vi "RT_Main.vi"(8 "ErrorIn":errorcluster, 11 "ClusterIn":T1={"MainQ"=refnum, "User"={"Lvl"=enum."Admin", "Pwd"=""}, "Stat"={"SysState"=enum."Init"}, "Paths"={"CfgFile"=path "", "LogFolder"=path "", "LogFile"=path ""}, "HW"={"HW?"=FALSE, "HWMode"=enum."HW_Init", "Refs"={"Visa"="GPIB0::2::INSTR"}}, "RTConfig"={"Arm"=FALSE, "Number"=0.0, "String"=""}}) -> (0 "ErrorOut":errorcluster, 3 "ClusterOut":T1={"MainQ"=refnum, "User"={"Lvl"=enum."Admin", "Pwd"=""}, "Stat"={"SysState"=enum."Init"}, "Paths"={"CfgFile"=path "", "LogFolder"=path "", "LogFile"=path ""}, "HW"={"HW?"=FALSE, "HWMode"=enum."HW_Init", "Refs"={"Visa"="GPIB0::2::INSTR"}}, "RTConfig"={"Arm"=FALSE, "Number"=0.0, "String"=""}})   [LabVIEW 2018]
doc: "This is the main application VI and is a good framework to begin all applications with. See block diagram for detailed documentation.\n\n\nCopyright © 2011 Epimedia, Inc. All Rights Reserved.\n\nThe Epimedia Application Library is Copyright © 2009-2011 Epimedia, Inc. \nAll Rights Reserved. Used under license."
uses:
  Controls/UserLevelEnum_RT.ctl
  Queue/RTMainQueueElements.ctl
  Queue/HWQueueElements.ctl
  Queue/HyperVisor.ctl
  Controls/SystemStateEnum_RT.ctl
  Controls/Enums/RT_WinRead_Enum_RT.ctl
  Controls/Clusts/StreamClust.ctl
  <resource>/objmgr/ni.dex.rc
  Controls/Enums/WriteStream_RT.ctl
  Queue/MainQueueElements.ctl
  Controls/RT_Config.ctl
  Controls/HWCluster_RT.ctl
  Controls/HWRefsCluster_RT.ctl
  Controls/MasterCluster_RT.ctl
  Controls/PathsCluster_RT.ctl
  Controls/UserCluster_RT.ctl
  Controls/SystemStatusCluster_RT.ctl
panel:
  out "30 Second Time":string
  out "CPU":dbl
  in  "ReInitHW":bool
  in  "ErrorIn":errorcluster
  out "Time":timestamp caption="Current Date/Time" format="%<%H:%M:%S%1u\n%m/%d/%Y>T"
  in  "Start":bool
  in  "Exit":bool
  in  "Stop":bool
  # "Copyright © 2011 Epimedia, Inc. All Rights Reserved.\n\nThe Epimedia Application Library is Copyright © 2009-2011 Epimedia, Inc. \nAll Rights Reserved. Used under license."
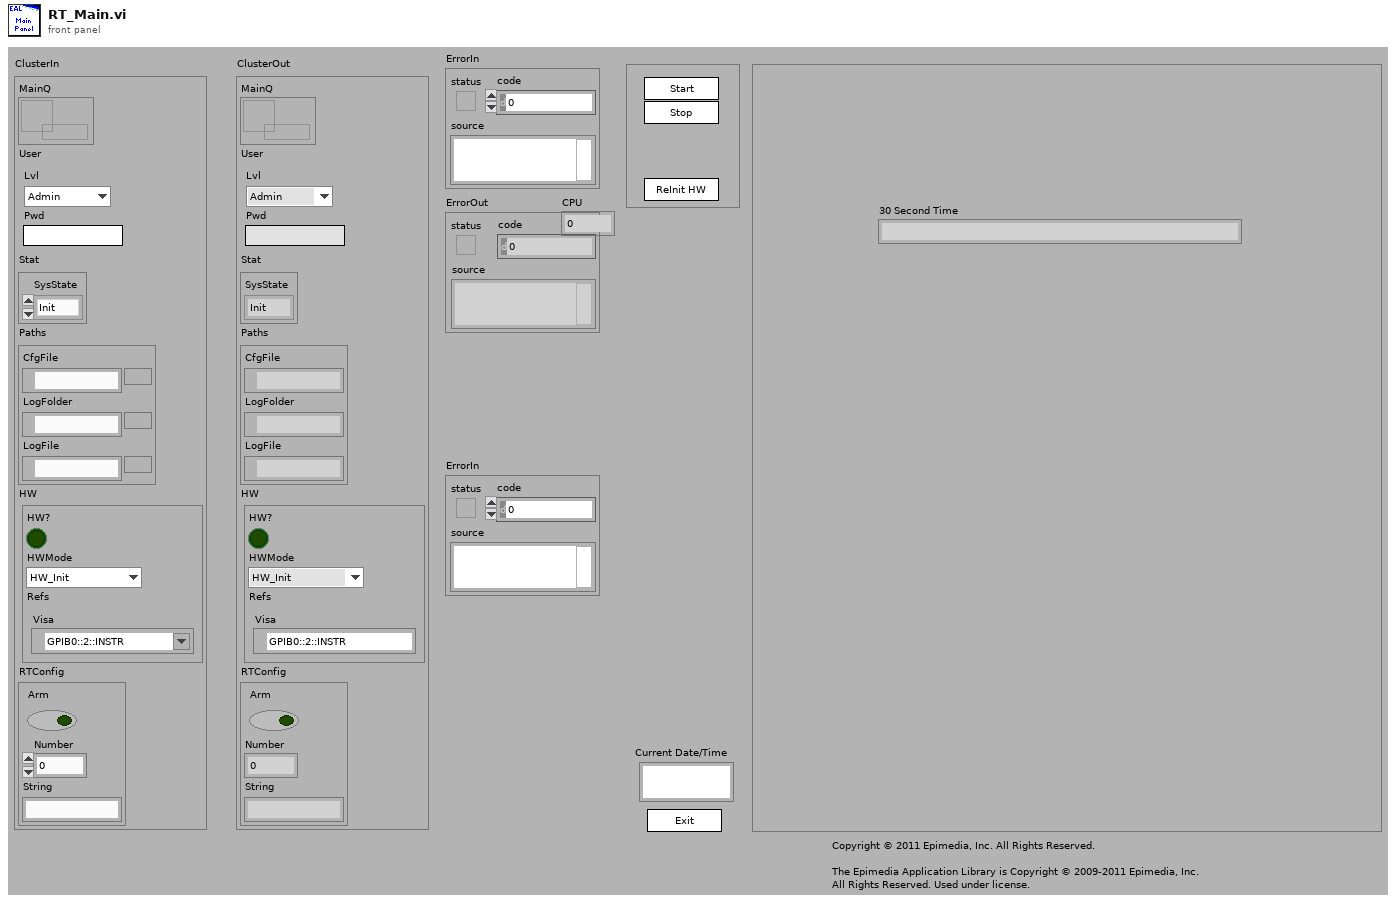
[diagram p1: front panel]
types:
  T1 = typedef "MasterCluster_RT.ctl" = cluster{"MainQ":refnum<queue>, "User":T2, "Stat":T4, "Paths":T6, "HW":T7, "RTConfig":T10}
  T2 = typedef "UserCluster_RT.ctl" = cluster{"Lvl":T3, "Pwd":string}
  T3 = typedef "UserLevelEnum_RT.ctl" = enum16{"Admin", "Operator"}
  T4 = typedef "SystemStatusCluster_RT.ctl" = cluster{"SysState":T5}
  T5 = typedef "SystemStateEnum_RT.ctl" = enum16{"Init", "Idle", "Running", "Error", "Exit"}
  T6 = typedef "PathsCluster_RT.ctl" = cluster{"CfgFile":path, "LogFolder":path, "LogFile":path}
  T7 = typedef "HWCluster_RT.ctl" = cluster{"HW?":bool, "HWMode":T8, "Refs":T9}
  T8 = typedef "HWQueueElements.ctl" = enum16{"HW_Init", "HW_UpdtCfg", "HW_Start", "HW_Pause", "HW_Run", "HW_Cls", "HW_Exit"}
  T9 = typedef "HWRefsCluster_RT.ctl" = cluster{"Visa":refnum<visa-resource-name>}
  T10 = typedef "RT_Config.ctl" = cluster{"Arm":bool, "Number":dbl, "String":string}
  T11 = typedef "WriteStream_RT.ctl" = enum16{"CreateWrtr", "SendStrm"}
  T12 = enum16{"open", "replace", "create", "open or create", "replace or create", "replace or create with confirmation"}
  T13 = typedef "RT_WinRead_Enum_RT.ctl" = enum16{"Init", "Read", "AUTO_Poll"}
  T14 = typedef "HyperVisor.ctl" = cluster{"TimeOut":dbl, string, "Data":variant, "StopHpvsr":bool}
  T15 = typedef "RTMainQueueElements.ctl" = enum16{"RTMain_InitQ", "RTMain_InitSW", "RTMain_InitCtrls", "RTMain_ReInitHW", "RTMain_FromStream", "RTMain_StrtHWLp", "RTMain_UpdtHWClstr", "RTMain_Start", "RTMain_Stop", "RTMain_Error", "RTMain_Config", "RTMain_Exit"}
  T16 = typedef "HWQueueElements.ctl" = enum16{"RTHW_Init", "RTHW_UpdtCfg", "RTHW_Start", "RTHW_Pause", "RTHW_Run", "RTHW_Cls", "RTHW_Exit"}
  T17 = typedef "MasterCluster.ctl" = cluster{"Admin":T18, "RTConfig":T10, "SMS":T20, "FPGA":T21, "Config":T23, "Stat":T33, "Alarm":T35}
  T18 = typedef "AdminCluster.ctl" = cluster{"Lvl":T19, "Pwd":string}
  T19 = typedef "UserLevelEnum.ctl" = enum16{"Admin", "Operator"}
  T20 = typedef "SMSDataCluster.ctl" = cluster{"Enbl?":bool, "Addr":string[]}
  T21 = typedef "FPGA_Config_Clust.ctl" = cluster{"Target":T22, "Channel":T22, "Ref1":refnum<k20>, "Ref2":refnum<k20>}
  T22 = typedef "TargetNumber.ctl" = enum16{"1", "2", "3", "4"}
  T23 = typedef "Config_Clust.ctl" = cluster{"UsrCfg":T24, "FP_User":T26}
  T24 = typedef "UserConfig.ctl" = cluster{"Paths":T25, "SampleRate":dbl}
  T25 = typedef "PathsCluster.ctl" = cluster{"CfgFile":path, "LogFolder":path, "LogFile":path, "NAS path":path, "ThreshFile":path, "RedunFolder":path}
  T26 = typedef "FrontPanel_UserConfig.ctl" = cluster{"#NoiseSums":u32, "Max_df":u32, "AvgAvg":bool, "#Avg":u16, "AutoCenter":bool, "Inclin":T27, "1":T28, "2":T28, "3":T28, "4":T28, "Target to Probe":T22, "SNR_Thresh":dbl, "Paths":T25, "Connex_Location":string, "SimulateFPGA":bool}
  T27 = typedef "Inclinometer_User_Cfg.ctl" = cluster{"Vmin":dbl, "Vmax":dbl, "Angle_min":dbl, "Angle_max":dbl, "Offset":dbl, "Pos_Neg":bool}
  T28 = typedef "FP_UserTargetConfig.ctl" = cluster{"Cal_":T29, "Beac":T29, "Scale":T30, "Offset":fxp<+/-,16,16>, "Scale_Noise":fxp<+/-,30,30>, "Scale_Step1":fxp<+/-,17,17>, "Scale_In_RT":ext, "ScaleMeas":fxp<+/-,16,1>, "FreqsToRemove":i32[], "Width":i32[], "ScaleMeasEnum":T31, "FilterEnab":T32}
  T29 = typedef "FreqShift.ctl" = cluster{"Fine":dbl, "Coarse_":dbl}
  T30 = typedef "FPGA_Scale.ctl" = cluster{"Step4":fxp<+/-,23,23>, "Step5":fxp<+/-,23,23>, "Step6":fxp<+/-,23,23>, "Step7":fxp<+/-,23,23>}
  T31 = typedef "ScaleMeasure.ctl" = enum16{"1", "10", "50", "42"}
  T32 = typedef "FilterEnableRadio.ctl" = enum32{"None", "Step 1", "Frequency Shift", "Step 4", "Step 5", "Step 6", "Step 7"}
  T33 = typedef "SystemStatusCluster.ctl" = cluster{"SysState":T34, "TrackRate":bool, "AutoCentr":bool}
  T34 = typedef "SystemStateEnum.ctl" = enum16{"Init", "Idle", "Running", "System Fault", "System Error", "Exit"}
  T35 = typedef "AlarmSettingsClust.ctl" = cluster{"TC13":T36, "AI1":T36, "AI2":T36, "AI3":T36, "AI4":T36, "AI5":T36, "AI6":T36, "AI18":T36, "AI19":T36, "TE1":T36, "TE2":T36, "TE3":T36, "ADAM1":T36, "ADAM2":T36, "ADAM3":T36, "ADAM4":T36, "72CoBeacFreq":T36, "72CoCalFreq":T36, "84CoBeacFreq":T36, "84CoCalFreq":T36, "72Co_CalTonePwr":T36, "72X_CalTonePwr":T36, "84Co_CalTonePwr":T36, "84X_CalTonePwr":T36}
  T36 = typedef "AlarmThresh_OneChan.ctl" = cluster{"Enbl":bool, "ErrsAndWarns":cluster{dbl, dbl, dbl, dbl}}
  T37 = typedef "MainQueueElements.ctl" = enum16{"Spvsr_InitQ", "Spvsr_RfrshPnl", "Spvsr_InitSW", "Spvsr_InitCtrls", "Spvsr_Cursors", "Spvsr_StrtHWLp", "Spvsr_Stop", "Spvsr_NewData", "Spvsr_ScaleGraphs", "Spvsr_Error", "Spvsr_About", "Spvsr_Config", "Spvsr_FPConfig", "Spvsr_AlarmCfg", "Spvsr_DigitzOffs", "FP_AO_ctrl", "Spvsr_RestartWarn", "Spvsr_AutoCenter", "Spvsr_TrackRate", "Spvsr_ChkTime", "Spvsr_Admin", "Spvsr_Exit"}
  T38 = typedef "NI_Real-Time Target Support.lvlib/RT CPU Load.ctl" = cluster{"Total (%)":dbl, "Time Critical (%)":dbl, "Timed Structures (%)":dbl, "High (%)":dbl, "Above Normal (%)":dbl, "Normal (%)":dbl, "Background (%)":dbl, "Idle (%)":dbl, "ISR (%)":dbl}
  T39 = typedef "StreamClust.ctl" = cluster{u16, variant}
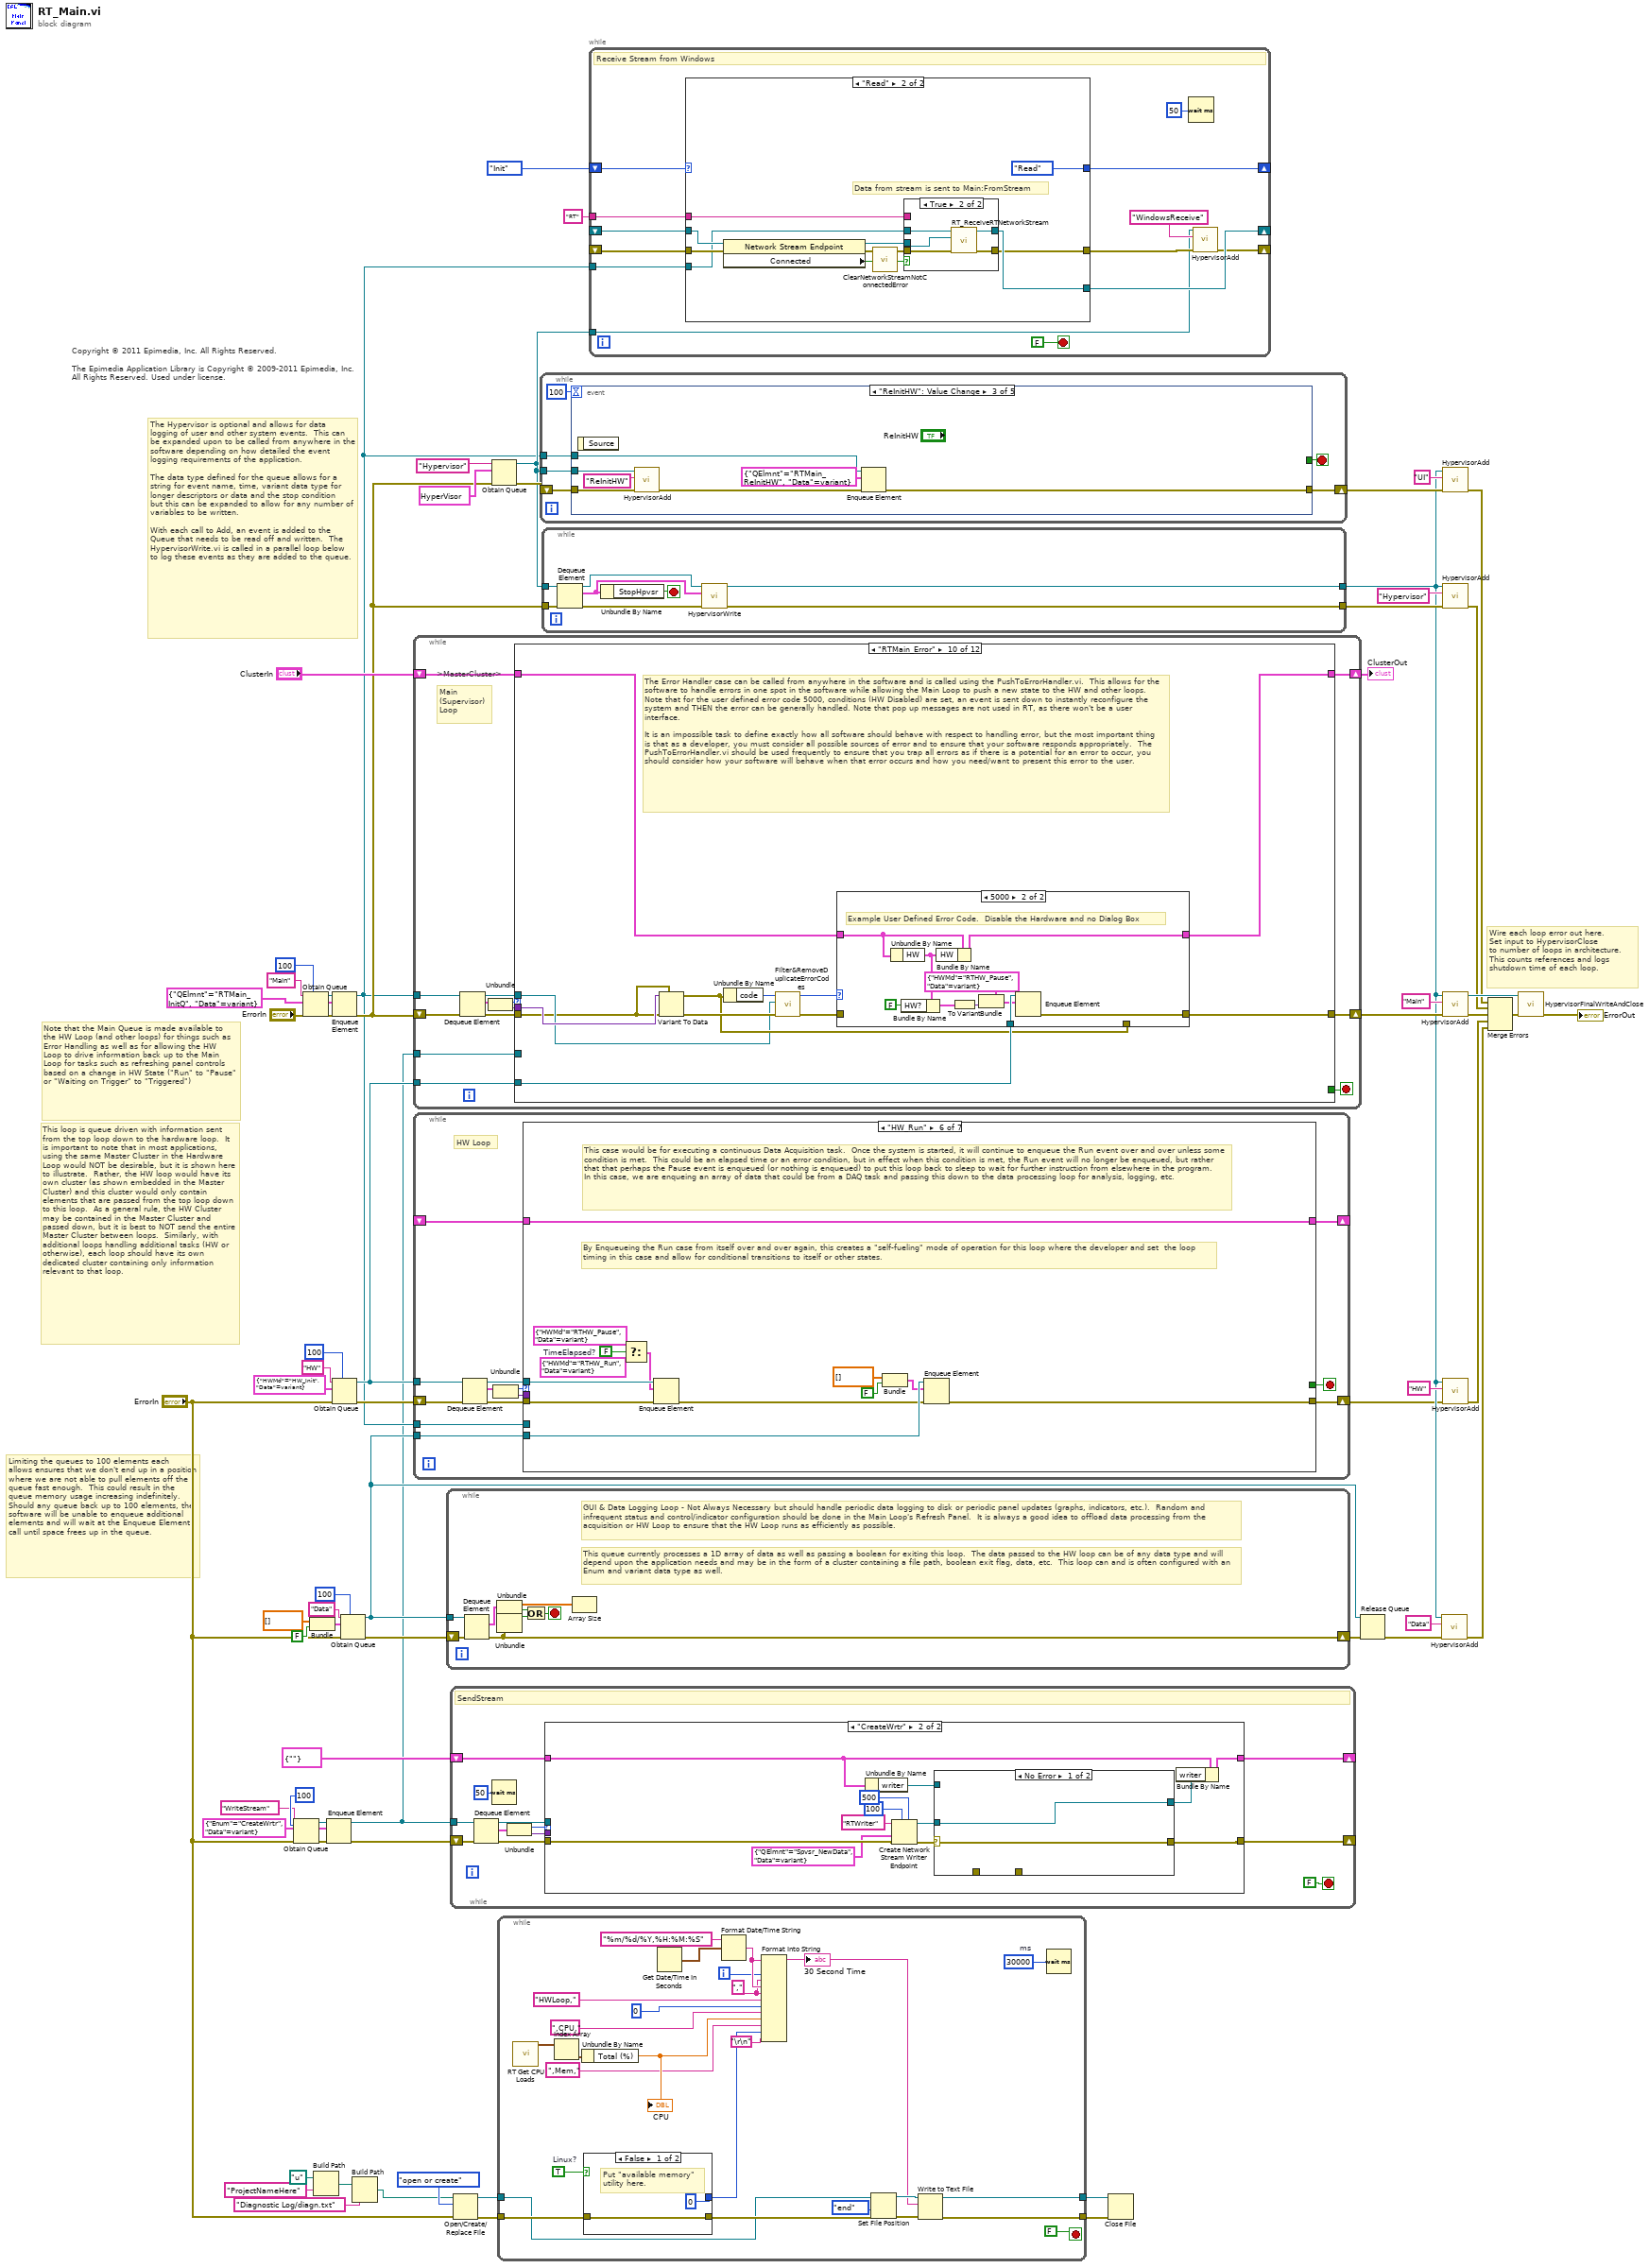
[diagram p0: block diagram]
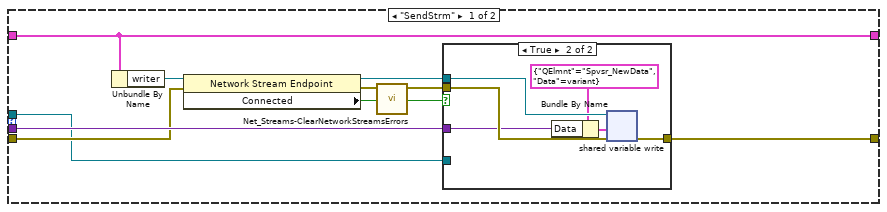
[diagram p2: hidden frame]
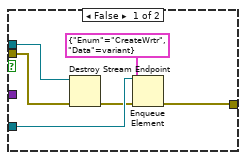
[diagram p3: hidden frame]
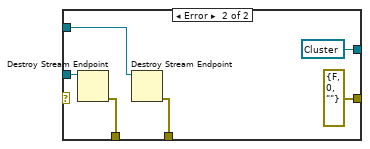
[diagram p4: hidden frame]
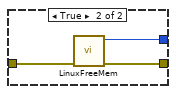
[diagram p5: hidden frame]
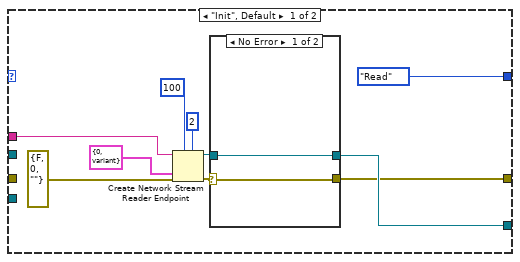
[diagram p6: hidden frame]
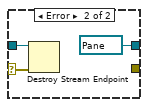
[diagram p7: hidden frame]
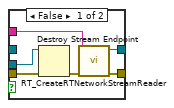
[diagram p8: hidden frame]
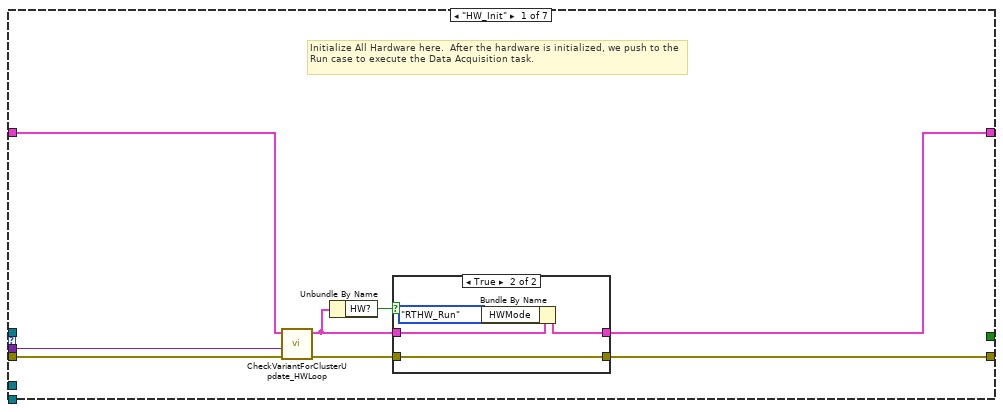
[diagram p9: hidden frame]
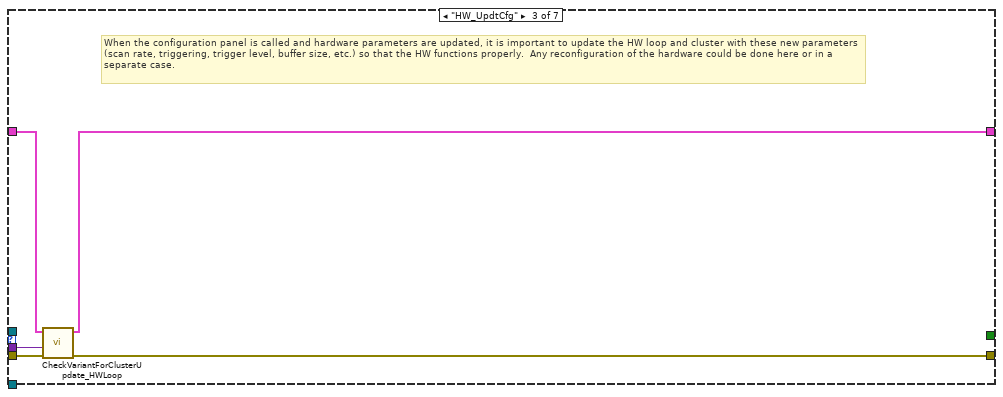
[diagram p12: hidden frame]
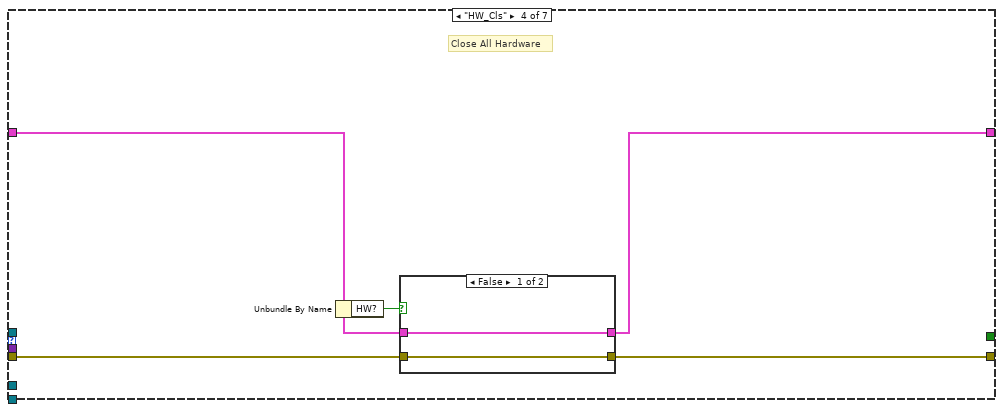
[diagram p13: hidden frame]
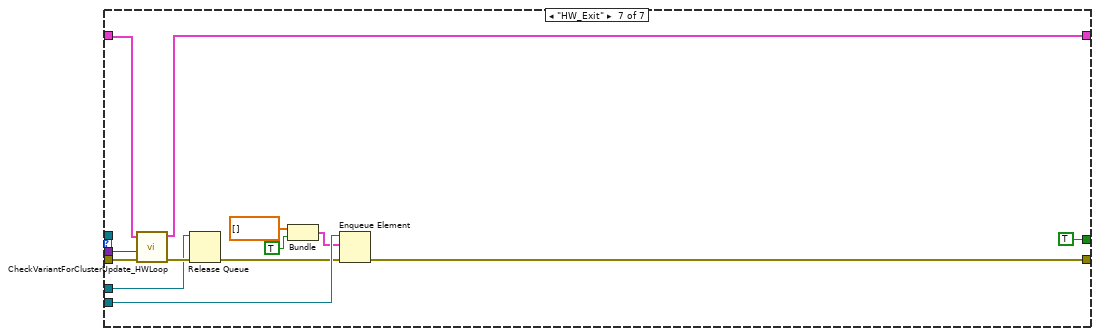
[diagram p16: hidden frame]
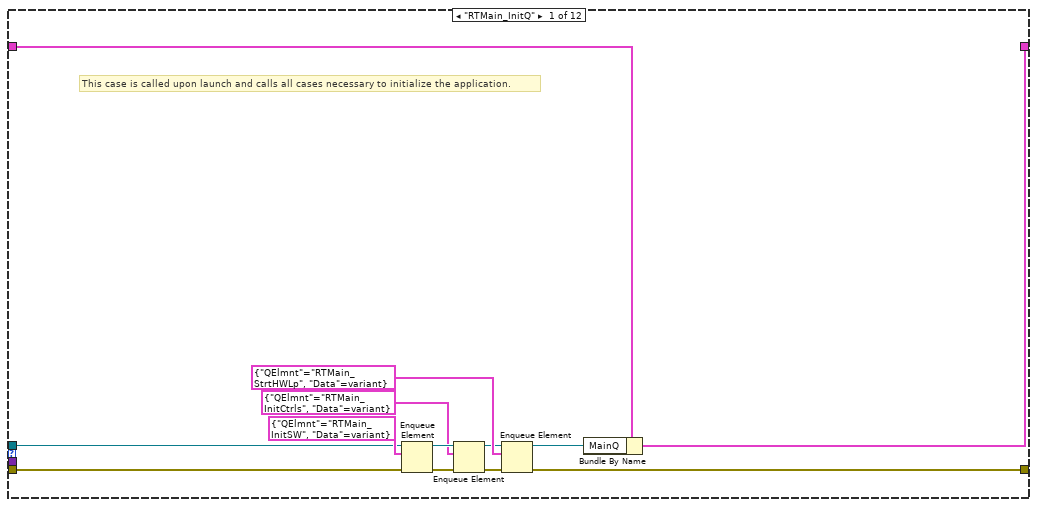
[diagram p17: hidden frame]
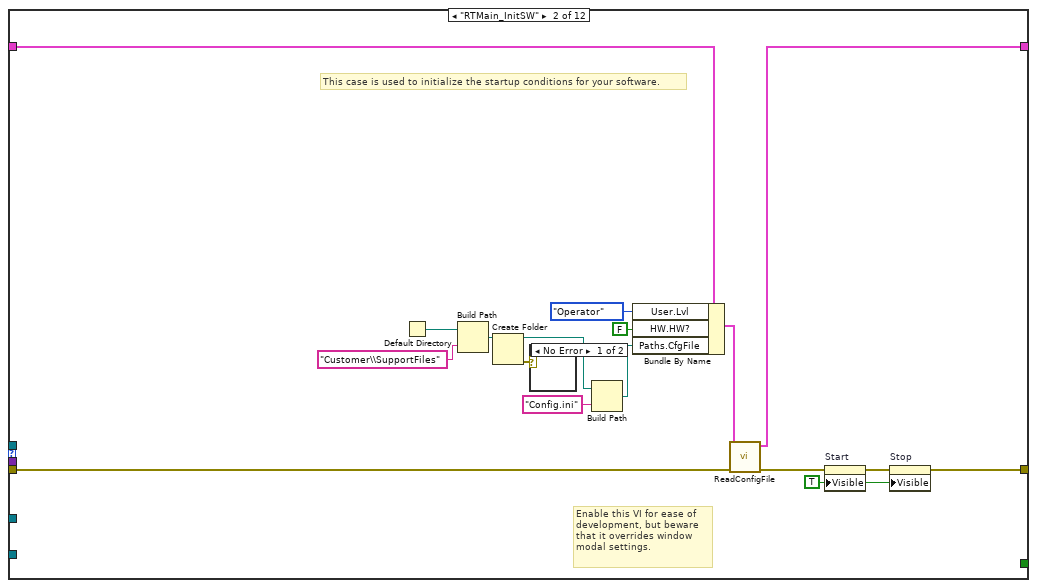
[diagram p18: hidden frame]
diagram:
  w12 = cluster{"Enum":T11, "Data":variant} {"Enum"=enum."CreateWrtr", "Data"=variant} ("output cluster")
  w62 = cluster{"QElmnt":T15, "Data":variant} {"QElmnt"=enum."RTMain_InitQ", "Data"=variant} ("Cluster")
  # "Note that the Main Queue is made available to the HW Loop (and other loops) for things such as Error Handling as well as for allowing the HW Loop to drive information back up to the Main Loop for tasks such as refreshing panel controls  based on a change in HW State (\"Run\" to \"Pause\" or \"Waiting on Trigger\" to \"Triggered\")"
  # "Limiting the queues to 100 elements each allows ensures that we don't end up in a position where we are not able to pull elements off the queue fast enough.  This could result in the queue memory usage increasing indefinitely.  Should any queue back up to 100 elements, the software will be unable to enqueue additional elements and will wait at the Enqueue Element call until space frees up in the queue."
  # "Wire each loop error out here.\nSet input to HypervisorClose\nto number of loops in architecture.\nThis counts references and logs\nshutdown time of each loop."
  # "The Hypervisor is optional and allows for data logging of user and other system events.  This can be expanded upon to be called from anywhere in the software depending on how detailed the event logging requirements of the application.\n\nThe data type defined for the queue allows for a string for event name, time, variant data type for longer descriptors or data and the stop condition but this can be expanded to allow for any number of variables to be written.\n\nWith each call to Add, an event is added to the Queue that needs to be read off and written.  The HypervisorWrite.vi is called in a parallel loop below to log these events as they are added to the queue."
  # "This loop is queue driven with information sent from the top loop down to the hardware loop.  It is important to note that in most applications, using the same Master Cluster in the Hardware Loop would NOT be desirable, but it is shown here to illustrate.  Rather, the HW loop would have its own cluster (as shown embedded in the Master Cluster) and this cluster would only contain elements that are passed from the top loop down to this loop.  As a general rule, the HW Cluster may be contained in the Master Cluster and passed down, but it is best to NOT send the entire Master Cluster between loops.  Similarly, with additional loops handling additional tasks (HW or otherwise), each loop should have its own dedicated cluster containing only information relevant to that loop."
  # "Copyright © 2011 Epimedia, Inc. All Rights Reserved.\n\nThe Epimedia Application Library is Copyright © 2009-2011 Epimedia, Inc. \nAll Rights Reserved. Used under license."
  n1 = Obtain Queue(max queue size (-1, unlimited)=100, name (unnamed)="WriteStream", element data type=w12, error in (no error)="ErrorIn") -> (queue out=w15:refnum<queue>, error out=w11:errorcluster)  [unwired: 1 in, 1 out]
  n2 = Obtain Queue(max queue size (-1, unlimited)=100, name (unnamed)="Main", element data type=w62, error in (no error)="ErrorIn") -> (queue out=w65:refnum<queue>, error out=w66:errorcluster)  [unwired: 1 in, 1 out]
  n3 = Bundle(dbl[] [], FALSE) -> (w27:cluster{dbl[], bool})  [unwired: 1 in]
  n4 = Build Path(base path=path "u", name or relative path="ProjectNameHere") -> (appended path=w3:path)
  n5 = Enqueue Element(queue=w15, element=w12, error in (no error)=w11) -> (queue out=w7:refnum<queue>, error out=w10:errorcluster)  [unwired: 1 in, 1 out]
  n6 = Enqueue Element(queue=w65, element=w62, error in (no error)=w66) -> (queue out=w8:refnum<queue>, error out=w40:errorcluster)  [unwired: 2 out]
  n7 = Obtain Queue(max queue size (-1, unlimited)=100, name (unnamed)="HW", element data type=cluster{"HWMd":T8, "Data":variant} {"HWMd"=enum."HW_Init", "Data"=variant}, error in (no error)="ErrorIn") -> (queue out=w31:refnum<queue>, error out=w30:errorcluster)  [unwired: 1 in, 1 out]
  n8 = Obtain Queue(max queue size (-1, unlimited)=100, name (unnamed)="Data", element data type=w27, error in (no error)="ErrorIn") -> (queue out=w56:refnum<queue>, error out=w16:errorcluster)  [unwired: 1 in, 1 out]
  n9 = Build Path(base path=w3, name or relative path="Diagnostic Log/diagn.txt") -> (appended path=w1:path)
  n10 = while {
    shift-right: [w71] -> w47
    shift-left: w40 -> [w68]
    tunnel: w8 -> [w70]
    shift-right: [w73] -> w64
    shift-left: "ClusterIn" -> [w80]
    tunnel: w31 -> [w72]
    tunnel: w7 -> [w69]
    stop <- w79 stop-if-true
    # ">MasterCluster>"
    # "Main \n(Supervisor)\nLoop"
    n11 = Dequeue Element(queue=w70, error in (no error)=w68) -> (queue out=w78:refnum<queue>, element=w76:cluster{"QElmnt":T15, "Data":variant}, error out=w77:errorcluster)  [unwired: 2 out]
    n12 = Unbundle(w76) -> ("QElmnt"=w75:T15, "Data"=w74:variant)
    n13 = case shown="\"RTMain_Error\"" w75 {
      tunnel: w77 -> [w89 w96 w111 w116 w130 w133 w139 w146 w156 w161 w197 w207]
      tunnel: [w92 w99 w112 w122 w123 w132 w140 w149 w158 w165 w191 w205] -> w73
      tunnel: w80 -> [w93 w106 w112 w113 w123 w132 w141 w154 w159 w166 w193 w205]
      tunnel: [_ _ _ _ _ _ _ _ _ _ _ TRUE] -> w79
      tunnel: [w81 w107 w111 w115 w127 w137 w143 w151 w156 w168 w198 w206] -> w71
      tunnel: w78 -> [w90 _ _ _ w126 _ _ _ _ w162 _ _]
      tunnel: w74 -> [_ _ _ _ w129 _ w144 _ _ w163 w194 _]
      tunnel: w72 -> [_ _ _ w114 _ w138 _ w150 _ w167 w200 w208]
      tunnel: w69 -> [_ _ _ _ _ _ _ _ _ _ w188 _]
      frame "RTMain_InitQ" {
        # "This case is called upon launch and calls all cases necessary to initialize the application."
        n14 = Enqueue Element(queue=w90, element=cluster{"QElmnt":T15, "Data":variant} {"QElmnt"=enum."RTMain_InitSW", "Data"=variant} ("Cluster"), error in (no error)=w89) -> (queue out=w84:refnum<queue>, error out=w87:errorcluster)  [unwired: 1 in, 1 out]
        n15 = Enqueue Element(queue=w84, element=cluster{"QElmnt":T15, "Data":variant} {"QElmnt"=enum."RTMain_InitCtrls", "Data"=variant} ("Cluster"), error in (no error)=w87) -> (queue out=w85:refnum<queue>, error out=w86:errorcluster)  [unwired: 1 in, 1 out]
        n16 = Enqueue Element(queue=w85, element=cluster{"QElmnt":T15, "Data":variant} {"QElmnt"=enum."RTMain_StrtHWLp", "Data"=variant} ("Cluster"), error in (no error)=w86) -> (queue out=w82:refnum<queue>, error out=w81:errorcluster)  [unwired: 1 in, 1 out]
        n17 = Bundle By Name(cluster=w93, "MainQ"=w82) -> (w92:T1)
      }
      frame "RTMain_InitSW" {
        w94 = TRUE ("Visible")
        # "Enable this VI for ease of\ndevelopment, but beware\nthat it overrides window \nmodal settings."
        # "This case is used to initialize the startup conditions for your software."
        n18 = Default Directory() -> (w95:path)
        n19 = Build Path(base path=w95, name or relative path="Customer\\SupportFiles") -> (appended path=w103:path)
        n20 = Create Folder(path (use dialog)=w103) -> (created path=w102:path, error out=w104:errorcluster)  [unwired: 2 in, 1 out]
        n21 = case shown="No Error" w104 {
          frame No Error {
          }
          frame Error {
          }
        }
        n22 = Build Path(base path=w102, name or relative path="Config.ini") -> (appended path=w100:path)
        n23 = Bundle By Name(cluster=w106, "User.Lvl"=UserLevelEnum_RT."Operator", "HW.HW?"=FALSE ("HW?"), "Paths.CfgFile"=w100) -> (w110:T1)
        n24 = call "ReadConfigFile.vi"("ErrorIn"=w96, "ClusterIn"=w110) -> ("ErrorOut"=w98:errorcluster, "ClusterOut"=w99:T17)  [unwired: 1 in, 7 out]
        n25 = property on="Start" class="Bool"(error in=w98, "Visible"=w94) -> (error out=w109:errorcluster)  [unwired: 1 in, 1 out]
        n26 = property on="Stop" class="Bool"(error in=w109, "Visible"=w94) -> (error out=w107:errorcluster)  [unwired: 1 in, 1 out]
      }
      frame "RTMain_InitCtrls" {
        # "This case is used to set the system startup state by updating front panel controls if desired.  Examples of this would be to clear graphs for first run and/or update controls with values loaded from the Config File in the InitSW case."
      }
      frame "RTMain_ReInitHW" {
        # "The ReInitHW state is a very important case to most applications involving hardware interfacing.  With dedicated hardware loops that can generate errors, those errors are sent to the Supervisor loop's Error case where instructions are sent down to put those loops to a standby state and instructions should be given to the user for how to remedy the error.  The operator is alerted in the Error case that an error has occured and Refresh Panel makes the ReInitHW button available.   When the ReInitHW button is pressed, this case should then Re-Initialize the lower loops to try and get the system to return to normal operation"
        n27 = Unbundle By Name(w113) -> ("HW"=w117:T7)
        n28 = To Variant(anything=w117) -> (Variant=w118:variant)
        n29 = Bundle(cluster=cluster{"HWMd":T8, "Data":variant} {"HWMd"=enum."HW_Init", "Data"=variant}, "Data"=w118) -> (w119:cluster{"HWMd":T8, "Data":variant})  [unwired: 1 in]
        n30 = Enqueue Element(queue=w114, element=w119, error in (no error)=w116) -> (error out=w115:errorcluster)  [unwired: 1 in, 2 out]
        n31 = Bundle By Name(cluster=w113, "Stat.SysState"=SystemStateEnum_RT."Init") -> (w122:T1)
      }
      frame "RTMain_FromStream" {
        # "Data from the incoming stream is enqueued here. Admittedly, this could be done with one less step if incoming data was enqueued directly in the \"Read\"\ncase in the \"Receive Stream from Windows\" loop rather than repackaging it and sending it first to this case. Sending to this intermediary case, though,\ncould be helpful if complex monitoring of incoming data is needed.\nLuke 3/30/2016"
        n32 = Variant To Data(error in=w130, type=cluster{"QElmnt":T15, "Data":variant} {"QElmnt"=enum."RTMain_InitQ", "Data"=variant} ("element"), Variant=w129) -> (data=w124:cluster{"QElmnt":T15, "Data":variant}, error out=w128:errorcluster)
        n33 = Enqueue Element(queue=w126, element=w124, error in (no error)=w128) -> (error out=w127:errorcluster)  [unwired: 1 in, 2 out]
      }
      frame "RTMain_StrtHWLp" {
        # "Starts the HW Loop and this should only be called once all Main Loop and Software Initialization has occurred to ensure that the HW Loop has the newest data to operate on."
        n34 = Unbundle By Name(w132) -> ("HW"=w131:T7)
        n35 = To Variant(anything=w131) -> (Variant=w134:variant)
        n36 = Bundle(cluster=cluster{"HWMd":T8, "Data":variant} {"HWMd"=enum."HW_Init", "Data"=variant}, "Data"=w134) -> (w135:cluster{"HWMd":T8, "Data":variant})  [unwired: 1 in]
        n37 = Enqueue Element(queue=w138, element=w135, error in (no error)=w133) -> (error out=w137:errorcluster)  [unwired: 1 in, 2 out]
      }
      frame "RTMain_UpdtHWClstr" {
        n38 = Unbundle By Name(w141) -> ("HW"=w145:T7)
        n39 = call "CheckVariantForClusterUpdate_HWLoop.vi"("ErrorIn"=w139, "VariantIn"=w144, "ClusterIn"=w145) -> ("ErrorOut"=w143:errorcluster, "ClusterOut"=w142:T7)  [unwired: 7 in]
        n40 = Bundle By Name(cluster=w141, "HW"=w142) -> (w140:T1)
      }
      frame "RTMain_Start" {
        # "The Log file path is created here, but may need to be passed to a data logging loop, the HW loop or elsewhere depending on the application."
        n41 = Unbundle By Name(w154) -> ("Paths.LogFolder"=w155:path)
        n42 = call "CreateLogFile.vi"("ErrorIn"=w146, "LogFolder"=w155) -> ("ErrorOut"=w152:errorcluster, "LogFile"=w153:path)  [unwired: 5 in, 3 out]
        n43 = Bundle By Name(cluster=w154, "Stat.SysState"=SystemStateEnum_RT."Running", "Paths.LogFile"=w153) -> (w149:T1)
        n44 = Enqueue Element(queue=w150, element=cluster{"HWMd":T16, "Data":variant} {"HWMd"=enum."RTHW_Start", "Data"=variant}, error in (no error)=w152) -> (error out=w151:errorcluster)  [unwired: 3 out]
      }
      frame "RTMain_Stop" {
        # "The Stop case would stop the execution of a currently running test.  The System State is updated and Refresh Panel is called so that the front panel controls can be configured for this state."
        n45 = Bundle By Name(cluster=w159, "Stat.SysState"=SystemStateEnum_RT."Idle") -> (w158:T1)
      }
      frame "RTMain_Error" {
        # "The Error Handler case can be called from anywhere in the software and is called using the PushToErrorHandler.vi.  This allows for the software to handle errors in one spot in the software while allowing the Main Loop to push a new state to the HW and other loops.  Note that for the user defined error code 5000, conditions (HW Disabled) are set, an event is sent down to instantly reconfigure the system and THEN the error can be generally handled. Note that pop up messages are not used in RT, as there won't be a user interface.\n\nIt is an impossible task to define exactly how all software should behave with respect to handling error, but the most important thing is that as a developer, you must consider all possible sources of error and to ensure that your software responds appropriately.  The PushToErrorHandler.vi should be used frequently to ensure that you trap all errors as if there is a potential for an error to occur, you should consider how your software will behave when that error occurs and how you need/want to present this error to the user."
        n46 = Variant To Data(error in=w161, type=w161, Variant=w163) -> (data=w164:errorcluster, error out=w169:errorcluster)
        n47 = Unbundle By Name(w164) -> ("code"=w171:i32)
        n48 = call "Filter&RemoveDuplicateErrorCodes.vi"("ErrorIn"=w169, "MainQIn"=w162, "ErrorCodeIn"=w171) -> ("ErrorOut"=w160:errorcluster, "ErrorCodeOut"=w170:i32)  [unwired: 6 in, 1 out]
        n49 = case shown="5000" w170 {
          tunnel: [w172 w177] -> w168
          tunnel: w166 -> [w173 w175]
          tunnel: [w173 w174] -> w165
          tunnel: w160 -> [w172 _]
          tunnel: w164 -> [_ _]
          tunnel: w167 -> [_ w182]
          frame Default {
            # "This is where you could put a feature to send an email or text message\nwhen an unknown error arises."
            # "Default Error Case handles all error codes undefined by this structure."
          }
          frame 5000 {
            # "Example User Defined Error Code.  Disable the Hardware and no Dialog Box"
            n50 = Unbundle By Name(w175) -> ("HW"=w176:T7)
            n51 = Bundle By Name(cluster=w176, "HW?"=FALSE) -> (w181:T7)
            n52 = Bundle By Name(cluster=w175, "HW"=w176) -> (w174:T1)
            n53 = To Variant(anything=w181) -> (Variant=w178:variant)
            n54 = Bundle(cluster=cluster{"HWMd":T16, "Data":variant} {"HWMd"=enum."RTHW_Pause", "Data"=variant}, "Data"=w178) -> (w180:cluster{"HWMd":T16, "Data":variant})  [unwired: 1 in]
            n55 = Enqueue Element(queue=w182, element=w180) -> (error out=w177:errorcluster)  [unwired: 1 in, 3 out]
          }
        }
      }
      frame "RTMain_Config" {
        # "Here we're immediately\nsending configuration\nsettings back to Windows\nto be sure that the settings\nwere received."
        # "This HW Cluster constant is used for demonstration only.   The developer should update this cluster with the appropriate fields and then update these fields accordingly before sending down to the HW Loop."
        n56 = Variant To Data(error in=w197, type=T10 {"Arm"=FALSE, "Number"=0.0, "String"=""} ("RTConfig"), Variant=w194) -> (data=w184:T10, error out=w196:errorcluster)
        n57 = Bundle By Name(cluster=w193, "RTConfig"=w184) -> (w191:T1)
        n58 = Unbundle By Name(w191) -> ("Paths.CfgFile"=w192:path)
        n59 = call "WriteConfigFile.vi"("ErrorIn"=w196, 10:w184, "ClusterIn"=w192) -> ("ErrorOut"=w190:errorcluster)  [unwired: 1 in, 7 out]
        n60 = To Variant(anything=w184) -> (Variant=w185:variant)
        n61 = Bundle By Name(cluster=cluster{"Enum":T11, "Data":variant} {"Enum"=enum."SendStrm", "Data"=variant} ("element"), "Data"=w185) -> (w186:cluster{"Enum":T11, "Data":variant})
        n62 = Enqueue Element(queue=w188, element=w186, error in (no error)=w190) -> (error out=w189:errorcluster)  [unwired: 3 out]
        n63 = To Variant(anything=T7 {"HW?"=FALSE, "HWMode"=enum."HW_Init", "Refs"={"Visa"="GPIB0::2::INSTR"}} ("HW")) -> (Variant=w202:variant)
        n64 = Bundle(cluster=cluster{"HWMd":T16, "Data":variant} {"HWMd"=enum."RTHW_UpdtCfg", "Data"=variant}, "Data"=w202) -> (w201:cluster{"HWMd":T16, "Data":variant})  [unwired: 1 in]
        n65 = Enqueue Element(queue=w200, element=w201, error in (no error)=w189) -> (error out=w198:errorcluster)  [unwired: 3 out]
      }
      frame "RTMain_Exit" {
        # "With the Exit Button, we exit this loop and push the HW Loop to close."
        n66 = Enqueue Element(queue=w208, element=cluster{"HWMd":T16, "Data":variant} {"HWMd"=enum."RTHW_Exit", "Data"=variant}, error in (no error)=w207) -> (error out=w206:errorcluster)  [unwired: 3 out]
      }
    }
  }
  "ClusterOut" <- w64
  n67 = while {
    shift-right: [w212] -> w26
    shift-left: w30 -> [w210]
    shift-right: [w222] -> _
    shift-left: _ -> [w217]
    tunnel: w56 -> [w221]
    tunnel: w31 -> [w220]
    tunnel: w8 -> [w211]
    stop <- w213 stop-if-true
    # "HW Loop"
    n68 = Dequeue Element(queue=w220, error in (no error)=w210) -> (queue out=w215:refnum<queue>, element=w219:cluster{"HWMd":T8, "Data":variant}, error out=w216:errorcluster)  [unwired: 2 out]
    n69 = Unbundle(w219) -> ("HWMd"=w218:T8, "Data"=w214:variant)
    n70 = case shown="\"HW_Run\"" w218 {
      tunnel: [w230 w237 w240 w244 w254 w263 w280] -> w212
      tunnel: [w229 w238 w239 w245 w253 w267 w275] -> w222
      tunnel: w217 -> [w223 w238 w241 w247 w253 w267 w276]
      tunnel: w216 -> [w227 w237 w243 w248 w254 w266 w278]
      tunnel: w221 -> [_ _ _ _ _ w265 w277]
      tunnel: w215 -> [_ _ _ _ _ w260 _]
      tunnel: w214 -> [w225 _ w242 _ _ _ w279]
      tunnel: [_ _ _ _ _ _ TRUE ("Exit?")] -> w213
      tunnel: w211 -> [_ _ _ _ _ _ w269]
      frame "HW_Init" {
        # "Initialize All Hardware here.  After the hardware is initialized, we push to the Run case to execute the Data Acquisition task."
        n71 = call "CheckVariantForClusterUpdate_HWLoop.vi"("ErrorIn"=w227, "VariantIn"=w225, "ClusterIn"=w223) -> ("ErrorOut"=w226:errorcluster, "ClusterOut"=w224:T7)  [unwired: 7 in]
        n72 = Unbundle By Name(w224) -> ("HW?"=w228:bool)
        n73 = case shown="True" w228 {
          tunnel: w226 -> [w231 w233]
          tunnel: [w231 w233] -> w230
          tunnel: [w232 w234] -> w229
          tunnel: w224 -> [w232 w236]
          frame False {
          }
          frame True {
            n74 = Bundle By Name(cluster=w236, "HWMode"=HWQueueElements."RTHW_Run" ("Stat.HWMd")) -> (w234:T7)
          }
        }
      }
      frame "HW_Start" {
        # "This case is where the acquisition task is to be started. An example would be to perhaps configure the DAQ task to use a Hardware Trigger to begin."
      }
      frame "HW_UpdtCfg" {
        # "When the configuration panel is called and hardware parameters are updated, it is important to update the HW loop and cluster with these new parameters (scan rate, triggering, trigger level, buffer size, etc.) so that the HW functions properly.  Any reconfiguration of the hardware could be done here or in a separate case."
        n75 = call "CheckVariantForClusterUpdate_HWLoop.vi"("ErrorIn"=w243, "VariantIn"=w242, "ClusterIn"=w241) -> ("ErrorOut"=w240:errorcluster, "ClusterOut"=w239:T7)  [unwired: 7 in]
      }
      frame "HW_Cls" {
        # "Close All Hardware"
        n76 = Unbundle By Name(w247) -> ("HW?"=w246:bool)
        n77 = case shown="False" w246 {
          tunnel: w248 -> [w249 w251]
          tunnel: [w249 w251] -> w244
          tunnel: [w250 w252] -> w245
          tunnel: w247 -> [w250 w252]
          frame False {
          }
          frame True {
          }
        }
      }
      frame "HW_Pause" {
      }
      frame "HW_Run" {
        w258 = FALSE  # TimeElapsed?
        # "By Enqueueing the Run case from itself over and over again, this creates a \"self-fueling\" mode of operation for this loop where the developer and set  the loop timing in this case and allow for conditional transitions to itself or other states."
        # "This case would be for executing a continuous Data Acquisition task.  Once the system is started, it will continue to enqueue the Run event over and over unless some condition is met.  This could be an elapsed time or an error condition, but in effect when this condition is met, the Run event will no longer be enqueued, but rather that that perhaps the Pause event is enqueued (or nothing is enqueued) to put this loop back to sleep to wait for further instruction from elsewhere in the program.  In this case, we are enqueing an array of data that could be from a DAQ task and passing this down to the data processing loop for analysis, logging, etc."
        n78 = Select(t=cluster{"HWMd":T16, "Data":variant} {"HWMd"=enum."RTHW_Pause", "Data"=variant} ("element"), s=w258, f=cluster{"HWMd":T16, "Data":variant} {"HWMd"=enum."RTHW_Run", "Data"=variant} ("element")) -> (s? t:f=w259:cluster{"HWMd":T16, "Data":variant})
        n79 = Enqueue Element(queue=w260, element=w259, error in (no error)=w266) -> (error out=w264:errorcluster)  [unwired: 3 out]
        n80 = Bundle(dbl[] [], FALSE) -> (w255:cluster{dbl[], bool})  [unwired: 1 in]
        n81 = Enqueue Element(queue=w265, element=w255, error in (no error)=w264) -> (error out=w263:errorcluster)  [unwired: 3 out]
      }
      frame "HW_Exit" {
        n82 = call "CheckVariantForClusterUpdate_HWLoop.vi"("ErrorIn"=w278, "VariantIn"=w279, "ClusterIn"=w276) -> ("ErrorOut"=w271:errorcluster, "ClusterOut"=w275:T7)  [unwired: 7 in]
        n83 = Release Queue(queue=w269, error in (no error)=w271) -> (error out=w270:errorcluster)  [unwired: 1 in, 2 out]
        n84 = Bundle(dbl[] [], TRUE) -> (w272:cluster{dbl[], bool})  [unwired: 1 in]
        n85 = Enqueue Element(queue=w277, element=w272, error in (no error)=w270) -> (error out=w280:errorcluster)  [unwired: 3 out]
      }
    }
  }
  n86 = while {
    shift-right: [w284] -> w57
    shift-left: w16 -> [w288]
    tunnel: w56 -> [w287]
    stop <- w286 stop-if-true
    # "This queue currently processes a 1D array of data as well as passing a boolean for exiting this loop.  The data passed to the HW loop can be of any data type and will depend upon the application needs and may be in the form of a cluster containing a file path, boolean exit flag, data, etc.  This loop can and is often configured with an Enum and variant data type as well."
    # "GUI & Data Logging Loop - Not Always Necessary but should handle periodic data logging to disk or periodic panel updates (graphs, indicators, etc.).  Random and infrequent status and control/indicator configuration should be done in the Main Loop's Refresh Panel.  It is always a good idea to offload data processing from the acquisition or HW Loop to ensure that the HW Loop runs as efficiently as possible."
    n87 = Dequeue Element(queue=w287, error in (no error)=w288) -> (element=w283:cluster{dbl[], bool}, error out=w284:errorcluster)  [unwired: 1 in, 2 out]
    n88 = Unbundle(w283) -> (w281:dbl[], w282:bool)
    n89 = Unbundle(w284) -> ("status"=w285:bool)  [unwired: 2 out]
    n90 = Or(x=w282, y=w285) -> (x .or. y?=w286:bool)
    n91 = Array Size(array=w281) -> ()  [unwired: 1 out]
  }
  n92 = while "Communication Loop" {
    shift-right: [w299] -> _
    shift-left: cluster{"writer":refnum<k21>} {"writer"=""} ("cluster") -> [w298]
    tunnel: w7 -> [w290]
    shift-right: [w289] -> _
    shift-left: w10 -> [w292]
    stop <- FALSE stop-if-true
    # "SendStream"
    n93 = Dequeue Element(queue=w290, error in (no error)=w292) -> (queue out=w293:refnum<queue>, element=w296:cluster{"Enum":T11, "Data":variant}, error out=w297:errorcluster)  [unwired: 1 in, 1 out]
    n94 = Wait (ms)(milliseconds to wait=u32 50) -> ()  [unwired: 1 out]
    n95 = Unbundle(w296) -> ("Enum"=w294:T11, "Data"=w295:variant)
    n96 = case shown="\"CreateWrtr\"" w294 {
      tunnel: [w309 w328] -> w289
      tunnel: [w310 w330] -> w299
      tunnel: w298 -> [w310 w326]
      tunnel: w293 -> [w301 _]
      tunnel: w297 -> [w306 w331]
      tunnel: w295 -> [w308 _]
      frame "SendStrm" {
        n97 = Unbundle By Name(w310) -> ("writer"=w304:refnum<k21>)
        n98 = property class="Network Stream Endpoint"(reference=w304, error in=w306) -> (reference out=w303:refnum<k21>, error out=w307:errorcluster, "Connected"=w302:bool)
        n99 = call "Net_Streams-ClearNetworkStreamsErrors.vi"("ErrorIn"=w307) -> ("ErrorOut"=w305:errorcluster)  [unwired: 10 in]
        n100 = case shown="True" w302 {
          tunnel: [w312 w322] -> w309
          tunnel: w308 -> [_ w319]
          tunnel: w305 -> [w315 w321]
          tunnel: w303 -> [w316 w320]
          tunnel: w301 -> [w314 _]
          frame False {
            n101 = Destroy Stream Endpoint(8:w315, 11:w316) -> (0:w313:errorcluster)
            n102 = Enqueue Element(queue=w314, element=cluster{"Enum":T11, "Data":variant} {"Enum"=enum."CreateWrtr", "Data"=variant} ("output cluster"), error in (no error)=w313) -> (error out=w312:errorcluster)  [unwired: 1 in, 2 out]
          }
          frame True {
            n103 = Bundle By Name(cluster=cluster{"QElmnt":T37, "Data":variant} {"QElmnt"=enum."Spvsr_NewData", "Data"=variant} ("Cluster"), "Data"=w319) -> (w318:cluster{"QElmnt":T37, "Data":variant})
            n104 = shared-variable-write(w320, w321, w318) -> (w322:errorcluster)  [unwired: 1 in, 2 out]
          }
        }
      }
      frame "CreateWrtr" {
        n105 = Unbundle By Name(w326) -> ("writer"=w325:refnum<k21>)
        n106 = Create Network Stream Writer Endpoint(5:500 ("timeout in ms (-1)"), 7:100 ("writer buffer size"), 8:w331, 9:cluster{"QElmnt":T37, "Data":variant} {"QElmnt"=enum."Spvsr_NewData", "Data"=variant} ("Cluster"), 11:"RTWriter" ("writer name")) -> (0:w334:errorcluster, 3:w324:refnum<k21>)  [unwired: 2 in]
        n107 = case shown="No Error" w334 {
          selector: w334 -> [w335 _]
          tunnel: w324 -> [w336 w342]
          tunnel: [w336 refnum<k21> refnum ("writer name")] -> w329
          tunnel: [w335 errorcluster {"status"=FALSE, "code"=0, "source"=""} ("error IO")] -> w328
          tunnel: w325 -> [_ w340]
          tunnel: [_ w339] -> _
          tunnel: [_ w338] -> _
          frame No Error {
          }
          frame Error {
            n108 = Destroy Stream Endpoint(11:w342) -> (0:w339:errorcluster)  [unwired: 1 in]
            n109 = Destroy Stream Endpoint(11:w340) -> (0:w338:errorcluster)  [unwired: 1 in]
          }
        }
        n110 = Bundle By Name(cluster=w326, "writer"=w329) -> (w330:cluster{"writer":refnum<k21>})
      }
    }
  }
  n111 = Open/Create/Replace File(file path (use dialog)=w1, error in="ErrorIn", operation (0:open)=T12."open or create") -> (refnum out=w18:refnum<file>, error out=w19:errorcluster)  [unwired: 4 out]
  n112 = Obtain Queue(name (unnamed)="Hypervisor", element data type=T14 {"TimeOut"=0.0, "", "Data"=variant, "StopHpvsr"=FALSE} ("HprVsr"), error in (no error)=w40) -> (queue out=w24:refnum<queue>, error out=w42:errorcluster)  [unwired: 2 in, 1 out]
  n113 = while {
    tunnel: w18 -> [w350]
    tunnel: w19 -> [w352]
    tunnel: [w354] -> w20
    tunnel: [w353] -> w21
    i -> [w345]
    stop <- FALSE stop-if-true
    w344 = TRUE  # Linux?
    w347 = u32 30000  # ms
    w346 = "," ("source")
    n114 = call <vilib>:"RT Get CPU Loads.vi"() -> ("CPU loads"=w359:T38[])  [unwired: 10 in, 1 out]
    n115 = Index Array(array=w359) -> (element=w358:T38)  [unwired: 1 in]
    n116 = Unbundle By Name(w358) -> ("Total (%)"=w357:dbl)
    "CPU" <- w357
    n117 = case shown="False" w344 {
      tunnel: w352 -> [w370 w373]
      tunnel: [w370 w372] -> w351
      tunnel: [u32 0 ("FreeMem") w371] -> w349
      frame False {
        # "Put \"available memory\"\nutility here."
      }
      frame True {
        n118 = call "LinuxFreeMem.vi"("error in"=w373) -> ("error out"=w372:errorcluster, "FreeMem"=w371:u32)  [unwired: 9 in]
      }
    }
    n119 = Get Date/Time In Seconds() -> (seconds since 1Jan1904=w364:timestamp)
    n120 = Format Date/Time String(time format string (%c)="%m/%d/%Y,%H:%M:%S", seconds (now)=w364) -> (date/time string=w362:string)  [unwired: 1 out]
    "30 Second Time" <- w362
    n121 = Format Into String(w345, w346, w362, w346, "HWLoop," ("source"), 0 ("input 6"), ",CPU," ("source"), w357, ",Mem," ("source"), w349, "\r\n") -> (resulting string=w365:string)  [unwired: 3 in, 1 out]
    n122 = Set File Position(refnum=w350, from (0:start)=enum16{"start", "end", "current"}."end", error in=w351) -> (refnum out=w367:refnum<file>, error out=w368:errorcluster)  [unwired: 1 out]
    n123 = Write to Text File(file (use dialog)=w367, text=w365, error in=w368) -> (refnum out=w354:refnum<file>, error out=w353:errorcluster)  [unwired: 2 out]
    n124 = Wait (ms)(milliseconds to wait=w347) -> ()  [unwired: 1 out]
  }
  n125 = while {
    tunnel: w8 -> [w378]
    shift-right: [w377] -> w53
    shift-left: w42 -> [w379]
    tunnel: w24 -> [w375]
    stop <- w376 stop-if-true
    n126 = event shown="[2] \"ReInitHW\": Value Change" {
      selector: _ -> [_ _ _ _ _]
      dyn-events: _ -> [_ _ _ _ _]
      timeout: 100 -> [_ _ _ _ _]
      tunnel: w379 -> [w381 w386 w393 w400 w407]
      tunnel: w378 -> [_ w387 w394 w401 w410]
      tunnel: [w381 w388 w395 w402 w409] -> w377
      tunnel: [_ _ _ _ TRUE] -> w376
      tunnel: w375 -> [_ w385 w392 w399 w406]
      event Timeout {
        # "Timeout Case is used to update 'heartbeat' clock on the front panel to provide an indication that the software is still running"
        n127 = event-data() -> ()  [unwired: 2 out]
        n128 = Get Date/Time In Seconds() -> (seconds since 1Jan1904=→"Time":timestamp)
      }
      event "Start": Value Change {
        n129 = event-data() -> ()  [unwired: 2 out]
        n130 = call "HypervisorAdd.vi"("ErrorIn"=w386, "ItemName"="Start", "QIn"=w385) -> ("ErrorOut"=w383:errorcluster)  [unwired: 7 in, 1 out]
        n131 = Enqueue Element(queue=w387, element=cluster{"QElmnt":T15, "Data":variant} {"QElmnt"=enum."RTMain_Start", "Data"=variant} ("Cluster"), error in (no error)=w383) -> (error out=w388:errorcluster)  [unwired: 3 out]
      }
      event "ReInitHW": Value Change {
        n132 = event-data() -> ()  [unwired: 2 out]
        n133 = call "HypervisorAdd.vi"("ErrorIn"=w393, "ItemName"="ReInitHW", "QIn"=w392) -> ("ErrorOut"=w390:errorcluster)  [unwired: 7 in, 1 out]
        n134 = Enqueue Element(queue=w394, element=cluster{"QElmnt":T15, "Data":variant} {"QElmnt"=enum."RTMain_ReInitHW", "Data"=variant} ("Cluster"), error in (no error)=w390) -> (error out=w395:errorcluster)  [unwired: 3 out]
      }
      event "Stop": Value Change {
        n135 = event-data() -> ()  [unwired: 2 out]
        n136 = call "HypervisorAdd.vi"("ErrorIn"=w400, "ItemName"="Stop", "QIn"=w399) -> ("ErrorOut"=w397:errorcluster)  [unwired: 7 in, 1 out]
        n137 = Enqueue Element(queue=w401, element=cluster{"QElmnt":T15, "Data":variant} {"QElmnt"=enum."RTMain_Stop", "Data"=variant} ("Cluster"), error in (no error)=w397) -> (error out=w402:errorcluster)  [unwired: 3 out]
      }
      event "Exit": Value Change; Panel Close {
        n138 = event-data() -> ()  [unwired: 2 out]
        n139 = call "HypervisorAdd.vi"("StopHpvsr"=TRUE, "ErrorIn"=w407, "ItemName"="Exit", "QIn"=w406) -> ("ErrorOut"=w404:errorcluster)  [unwired: 6 in, 1 out]
        n140 = Enqueue Element(queue=w410, element=cluster{"QElmnt":T15, "Data":variant} {"QElmnt"=enum."RTMain_Exit", "Data"=variant} ("Cluster"), error in (no error)=w404) -> (error out=w409:errorcluster)  [unwired: 3 out]
      }
    }
  }
  n141 = while {
    tunnel: w24 -> [w418]
    tunnel: w40 -> [w419]
    tunnel: [w417] -> w38
    tunnel: [w416] -> w37
    stop <- w413 stop-if-true
    n142 = Dequeue Element(queue=w418, error in (no error)=w419) -> (queue out=w415:refnum<queue>, element=w414:T14, error out=w412:errorcluster)  [unwired: 2 out]
    n143 = Unbundle By Name(w414) -> ("StopHpvsr"=w413:bool)
    n144 = call "HypervisorWrite.vi"("ErrorIn"=w412, "EventToLog"=w414, "QIn"=w415) -> ("ErrorOut"=w417:errorcluster, "QOut"=w416:refnum<queue>)  [unwired: 7 in]
  }
  n145 = while {
    tunnel: w24 -> [w421]
    shift-right: [w423] -> _
    shift-left: _ -> [w430]
    shift-right: [w427] -> _
    shift-left: RT_WinRead_Enum_RT."Init" ("Enum") -> [w429]
    shift-right: [w428] -> _
    shift-left: _ -> [w431]
    tunnel: "RT" ("SlaveName") -> [w425]
    tunnel: w8 -> [w420]
    stop <- FALSE stop-if-true
    # "Receive Stream from Windows"
    n146 = case shown="\"Read\"" w429 {
      tunnel: w420 -> [_ w451]
      tunnel: w431 -> [_ w453]
      tunnel: w430 -> [_ w455]
      tunnel: [w437 w449] -> w424
      tunnel: [RT_WinRead_Enum_RT."Read" ("Enum") RT_WinRead_Enum_RT."Read" ("Enum")] -> w427
      tunnel: [w439 w454] -> w428
      tunnel: w425 -> [w436 w450]
      frame "Init", Default {
        n147 = Create Network Stream Reader Endpoint(5:2 ("timeout in ms (-1)"), 7:100 ("reader buffer size"), 8:errorcluster {"status"=FALSE, "code"=0, "source"=""} ("error in (no error)"), 9:T39 {0, variant}, 11:w436) -> (0:w438:errorcluster, 3:w440:refnum<k21>)  [unwired: 2 in]
        n148 = case shown="No Error" w438 {
          selector: w438 -> [w443 w447]
          tunnel: [w443 _] -> w437
          tunnel: w440 -> [w444 w446]
          tunnel: [w444 refnum<k21> refnum ("SlaveName")] -> w439
          frame No Error {
          }
          frame Error {
            n149 = Destroy Stream Endpoint(8:w447, 11:w446) -> ()  [unwired: 1 out]
          }
        }
      }
      frame "Read" {
        # "Data from stream is sent to Main:FromStream"
        n150 = property class="Network Stream Endpoint"(reference=w453, error in=w455) -> (reference out=w458:refnum<k21>, error out=w456:errorcluster, "Connected"=w452:bool)
        n151 = call "ClearNetworkStreamNotConnectedError.vi"("ErrorIn"=w456) -> ("ErrorOut"=w457:errorcluster)  [unwired: 10 in]
        n152 = case shown="True" w452 {
          tunnel: w457 -> [w463 w468]
          tunnel: w451 -> [_ w467]
          tunnel: [w464 w469] -> w449
          tunnel: w458 -> [w461 w466]
          tunnel: [w460 w465] -> w454
          tunnel: w450 -> [w459 _]
          frame False {
            n153 = Destroy Stream Endpoint(8:w463, 11:w461) -> (0:w462:errorcluster)
            n154 = call "RT_CreateRTNetworkStreamReader.vi"("ErrorIn"=w462, "RT Stream Name"=w459) -> ("ErrorOut"=w464:errorcluster, "UI Stream Name"=w460:refnum<k21>)  [unwired: 8 in]
          }
          frame True {
            n155 = call "RT_ReceiveRTNetworkStream.vi"("ErrorIn"=w468, "Reader in"=w466, "queue"=w467) -> ("ErrorOut"=w469:errorcluster, "endpoint out"=w465:refnum<k21>)  [unwired: 7 in]
          }
        }
      }
    }
    n156 = Wait (ms)(milliseconds to wait=u32 50) -> ()  [unwired: 1 out]
    n157 = call "HypervisorAdd.vi"("ErrorIn"=w424, "ItemName"="WindowsReceive" ("LoopName"), "QIn"=w421) -> ("ErrorOut"=w423:errorcluster)  [unwired: 7 in, 1 out]
  }
  n158 = Close File(refnum=w20, error in=w21) -> ()  [unwired: 2 out]
  n159 = Release Queue(queue=w56, error in (no error)=w57) -> (error out=w49:errorcluster)  [unwired: 1 in, 2 out]
  n160 = call "HypervisorAdd.vi"("ErrorIn"=w49, "ItemName"="Data", "QIn"=w37) -> ("ErrorOut"=w43:errorcluster)  [unwired: 7 in, 1 out]
  n161 = call "HypervisorAdd.vi"("ErrorIn"=w53, "ItemName"="UI", "QIn"=w37) -> ("ErrorOut"=w36:errorcluster)  [unwired: 7 in, 1 out]
  n162 = call "HypervisorAdd.vi"("ErrorIn"=w38, "ItemName"="Hypervisor", "QIn"=w37) -> ("ErrorOut"=w35:errorcluster)  [unwired: 7 in, 1 out]
  n163 = call "HypervisorAdd.vi"("ErrorIn"=w47, "ItemName"="Main", "QIn"=w37) -> ("ErrorOut"=w46:errorcluster, "QOut"=w45:refnum<queue>)  [unwired: 7 in]
  n164 = call "HypervisorAdd.vi"("ErrorIn"=w26, "ItemName"="HW", "QIn"=w37) -> ("ErrorOut"=w44:errorcluster)  [unwired: 7 in, 1 out]
  n165 = Merge Errors(w36, w35, w46, w44, w43) -> (w41:errorcluster)
  n166 = call "HypervisorFinalWriteAndClose.vi"("ErrorIn"=w41, "QIn"=w45) -> ("ErrorOut"=→"ErrorOut":errorcluster)  [unwired: 9 in]
